vi "prepare_keyboard_notes.vi"(7 "Anticlockwise rotations [0-3] (0)":i32, 8 "error in (no error)":errorcluster, 9 "Note Length (-1)":dbl=-1.0, 10 "Total Length (1200)":dbl=1200.0, 11 "midi-ui in":refnum<class "midi-ui.lvclass">) -> (0 "error out":errorcluster, 3 "midi-ui out":refnum<class "midi-ui.lvclass">)   [LabVIEW 2020, in "midi-ui.lvclass"]
uses:
  midi-ui.lvclass
  midi-ui.lvclass/midi-ui.ctl
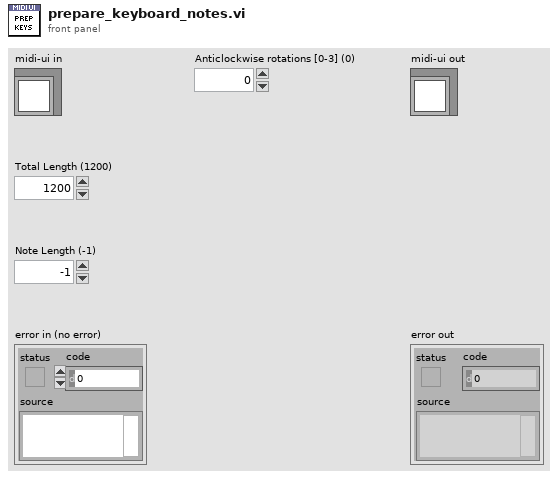
[diagram p1: front panel]
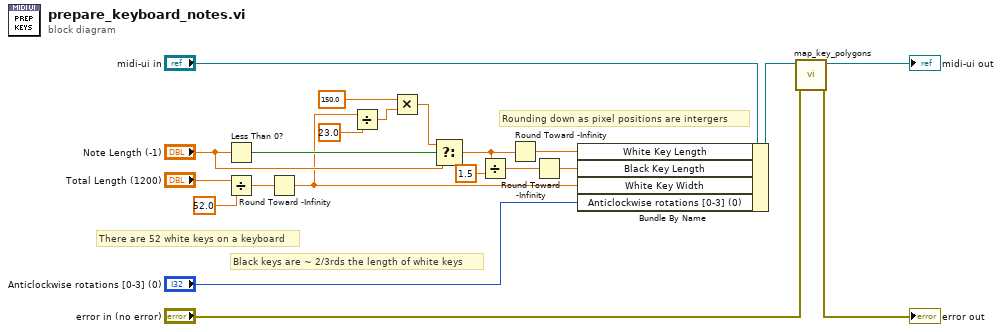
[diagram p0: block diagram]
diagram:
  # "Rounding down as pixel positions are intergers"
  # "Black keys are ~ 2/3rds the length of white keys"
  # "There are 52 white keys on a keyboard"
  n1 = Less Than 0?(x="Note Length (-1)") -> (x < 0?=w13:bool)
  n2 = Divide(x="Total Length (1200)", y=52.0) -> (x/y=w6:dbl)
  n3 = Round Toward -Infinity(1:w6) -> (0:w5:dbl)
  n4 = Divide(x=w5, y=23.0) -> (x/y=w10:dbl)
  n5 = Multiply(x=150.0 ("y"), y=w10) -> (x*y=w8:dbl)
  n6 = Select(t=w8, s=w13, f="Note Length (-1)") -> (s? t:f=w4:dbl)
  n7 = Divide(x=w4, y=1.5) -> (x/y=w2:dbl)
  n8 = Round Toward -Infinity(1:w4) -> (0:w3:dbl)
  n9 = Round Toward -Infinity(1:w2) -> (0:w1:dbl)
  n10 = Bundle By Name(cluster="midi-ui in", "White Key Length"=w3, "Black Key Length"=w1, "White Key Width"=w5, "Anticlockwise rotations [0-3] (0)"="Anticlockwise rotations [0-3] (0)") -> (w18:refnum<class "midi-ui.lvclass">)
  n11 = call "map_key_polygons.vi"("error in (no error)"="error in (no error)", "midi-ui in"=w18) -> ("error out"=→"error out":errorcluster, "midi-ui out"=→"midi-ui out":refnum<class "midi-ui.lvclass">)  [unwired: 8 in]
